vi "Set Image by ImagelistIndex.vi"(8 "error in (no error)":errorcluster caption="错误输入（无错误）", 10 "ImageIndex":i32, 11 "ToolStripLabel 输入":refnum<class "ToolStripLabel.lvclass"> caption="DNL_LabVIEW Object in") -> (0 "error out":errorcluster caption="错误输出", 3 "ToolStripLabel 输出":refnum<class "ToolStripLabel.lvclass"> caption="DNL_LabVIEW Object out")   [LabVIEW 2013, in "ToolStripLabel.lvclass"]
uses:
  ToolStripLabel.lvclass
  ToolStripLabel.lvclass/ToolStripLabel.ctl
  System.Windows.Forms
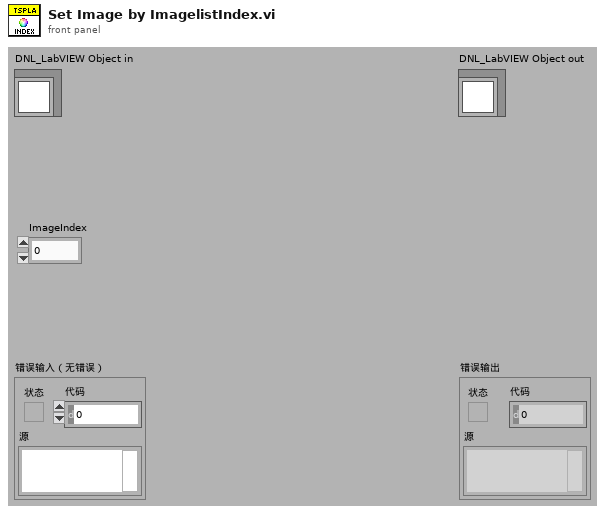
[diagram p1: front panel]
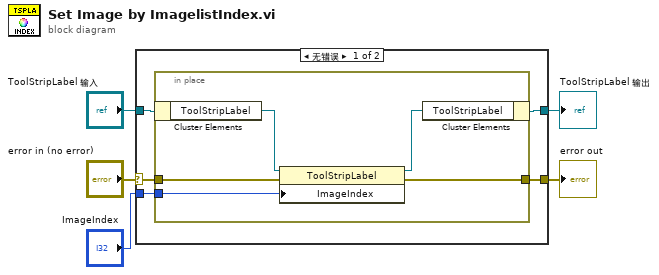
[diagram p0: block diagram]
diagram:
  n1 = case shown="无错误" "error in (no error)" {
    selector: "error in (no error)" -> [w8 w17]
    tunnel: [w7 w17] -> w4
    tunnel: [w6 w16] -> w2
    tunnel: "ToolStripLabel 输入" -> [w10 w16]
    tunnel: "ImageIndex" -> [w9 _]
    frame No Error {
      n2 = in-place {
        in-place-border: w9 -> [w13]
        in-place-border: w8 -> [w12]
        in-place-border: [w11] -> w7
        n3 = in-place-cluster #1(w10) -> ("ToolStripLabel"=w15:refnum<k24>)
        n4 = property class="ToolStripLabel"(reference=w15, error in=w12, "ImageIndex"=w13) -> (reference out=w14:refnum<k24>, error out=w11:errorcluster)
        n5 = in-place-cluster #1("ToolStripLabel"=w14) -> (w6:refnum<class "ToolStripLabel.lvclass">)
      }
    }
    frame Error {
    }
  }
  "error out" <- w4
  "ToolStripLabel 输出" <- w2
